vi "Initialize FINS.vi"(8 "error in (no error)":errorcluster) -> (0 "error out":errorcluster)   [LabVIEW 2016, in "Impedance Data Acquisition and Decoding.lvlib"]
doc: "Generates Initialization Sequence for FINS (1. Initialize Parameters 2. Alg cmd 3. Nav cmd)\n_____\nCreated using Delacor QMH Event Scripter 5.0.0.112."
uses:
  Impedance Data Acquisition and Decoding.lvlib
  Initialize FINS Argument--cluster.ctl
panel:
  in  "Init Alg Parameters":bool
  in  "Start Navigation":bool
  in  "Start Alignment":bool
  in  "Alignment Time":u8
  in  "Altitude":dbl
  in  "Longitude":dbl
  in  "Latitude":dbl
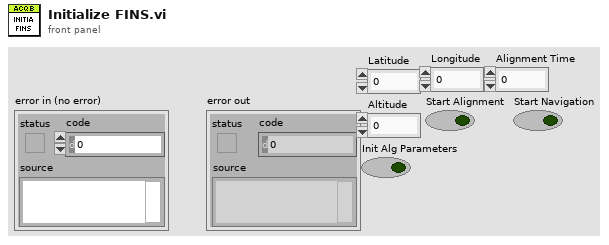
[diagram p1: front panel]
types:
  T1 = typedef "Impedance Data Acquisition and Decoding.lvlib/Initialize FINS Argument--cluster.ctl" = cluster{"Boolean":bool}
  T2 = typedef "Impedance Data Acquisition and Decoding.lvlib/Request Events--cluster.ctl" = cluster{"Stop Module":refnum<user-event>, "Show Panel":refnum<user-event>, "Hide Panel":refnum<user-event>, "Get Module Execution Status":refnum<user-event>, "Show Diagram":refnum<user-event>, "Stop Acquiring":refnum<user-event>, "Change Settings":refnum<user-event>, "Start Acquiring":refnum<user-event>, "WakeUp Helper Loop":refnum<user-event>, "Initialize FINS":refnum<user-event>, "Initialize FINS for FTR":refnum<user-event>, "Initialize FINS for Qualification":refnum<user-event>}
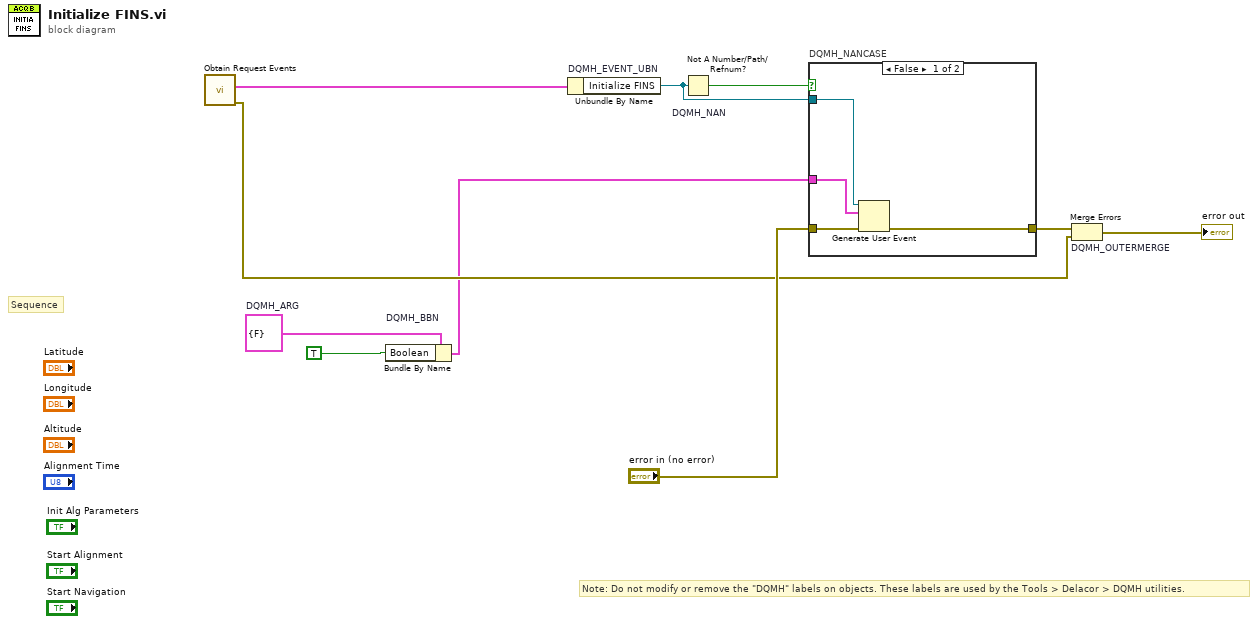
[diagram p0: block diagram]
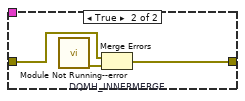
[diagram p2: hidden frame]
diagram:
  w5 = T1 {"Boolean"=FALSE}  # DQMH_ARG
  # "Sequence"
  # "Note: Do not modify or remove the \"DQMH\" labels on objects. These labels are used by the Tools > Delacor > DQMH utilities."
  n1 = call "Obtain Request Events.vi"() -> ("error out"=w3:errorcluster, "FINS3-E BusB Data Acquisition and Decoding Request Events"=w2:T2)  [unwired: 10 in]
  n2 = Bundle By Name "DQMH_BBN"(cluster=w5, "Boolean"=TRUE) -> (w1:T1)
  n3 = Unbundle By Name "DQMH_EVENT_UBN"(w2) -> ("Initialize FINS"=w7:refnum<user-event>)
  n4 = Not A Number/Path/Refnum? "DQMH_NAN"(number/path/refnum=w7) -> (NaN/Path/Refnum?=w8:bool)
  n5 = case "DQMH_NANCASE" shown="False" w8 {
    tunnel: "error in (no error)" -> [w14 w17]
    tunnel: [w13 w16] -> w6
    tunnel: w7 -> [w12 _]
    tunnel: w1 -> [w11 _]
    frame False {
      n6 = Generate User Event(user event=w12, event data cluster=w11, error in=w14) -> (error out=w13:errorcluster)  [unwired: 1 in, 1 out]
    }
    frame True {
      n7 = call "Module Not Running--error.vi"() -> ("error out"=w15:errorcluster)  [unwired: 11 in]
      n8 = Merge Errors "DQMH_INNERMERGE"(w17, w15) -> (w16:errorcluster)
    }
  }
  n9 = Merge Errors "DQMH_OUTERMERGE"(w6, w3) -> (→"error out":errorcluster)
